vi "Read Simulteneous.vi"(8 "error in (no error)":errorcluster, 11 "Scheduile Array in":refnum<class "Scheduile Array.lvclass">) -> (0 "error out":errorcluster, 2 "Simulteneous":bool=TRUE, 3 "Scheduile Array out":refnum<class "Scheduile Array.lvclass">)   [LabVIEW 2015, in "Scheduile Array.lvclass"]
uses:
  Scheduile Array.lvclass
  Scheduile Array.lvclass/Scheduile Array.ctl
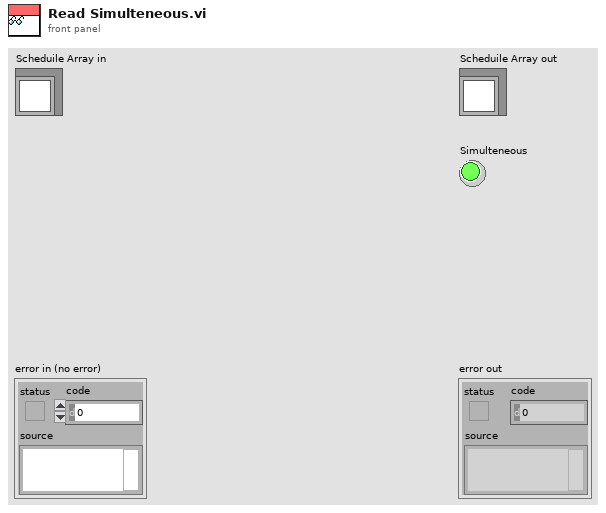
[diagram p1: front panel]
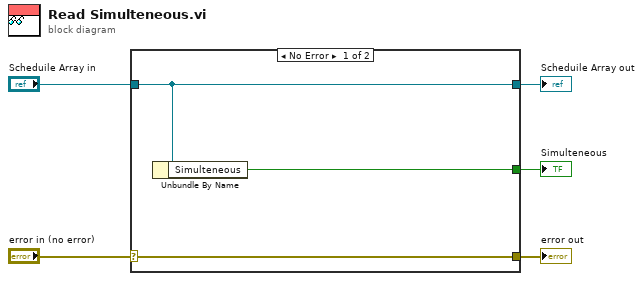
[diagram p0: block diagram]
diagram:
  n1 = case shown="No Error" "error in (no error)" {
    selector: "error in (no error)" -> [w8 w9]
    tunnel: [w8 w9] -> w4
    tunnel: [w7 w10] -> w2
    tunnel: "Scheduile Array in" -> [w7 w10]
    tunnel: [w6 _] -> w1
    frame No Error {
      n2 = Unbundle By Name(w7) -> ("Simulteneous"=w6:bool)
    }
    frame Error {
    }
  }
  "error out" <- w4
  "Scheduile Array out" <- w2
  "Simulteneous" <- w1
